vi "获取图像.vi"(1 "确定按钮":bool, 2 "File Path":path=path "C:/labview/labview_小米伺服_CAN总线/种子图片/2.jpeg", 3 "Session In":T1="cam6") -> (0 "Image":T2(plugin-control))   [LabVIEW 2023]
uses:
  <vilib>/userDefined/High Color/IMAQdx.ctl
  <vilib>/vision/driver/NI_Vision_Acquisition_Software.lvlib
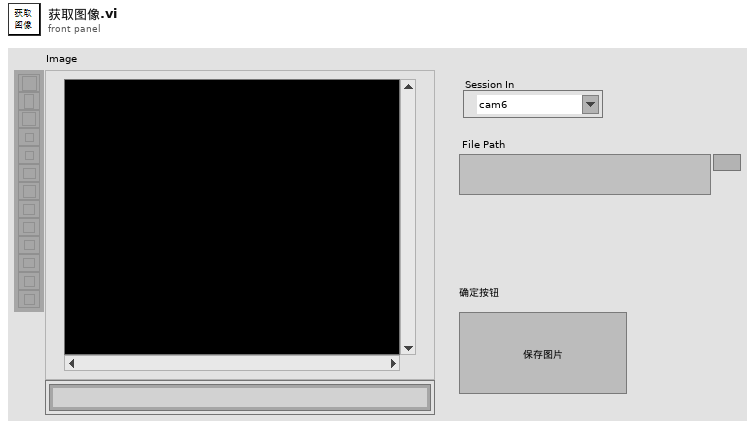
[diagram p1: front panel]
types:
  T1 = typedef "IMAQdx.ctl" = refnum<k21>
  T2 = typedef "IMAQ Image.ctl" = refnum<image>
  T3 = typedef "Image Type" = u32
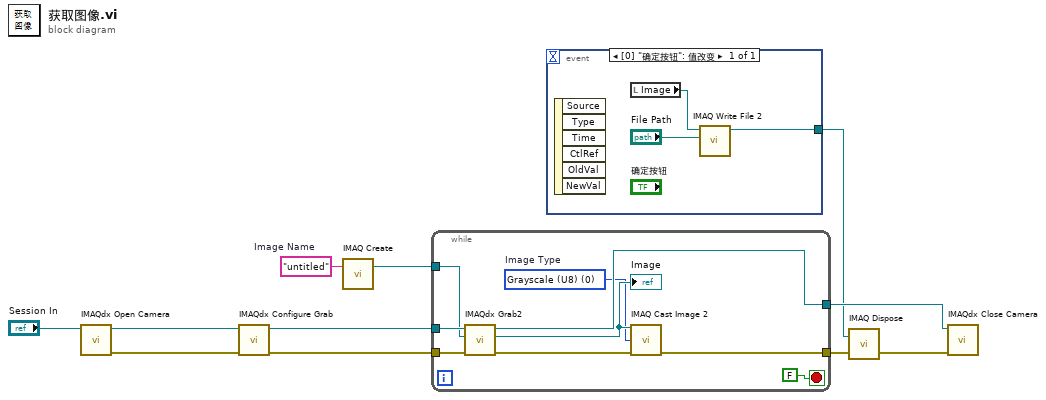
[diagram p0: block diagram]
diagram:
  w11 = "untitled"  # Image Name
  n1 = call <vilib>:"IMAQdx Open Camera.vi"("Session In"="Session In") -> ("error out"=w5:errorcluster, "Session Out"=w6:T1)  [unwired: 9 in]
  n2 = call <vilib>:"IMAQdx Configure Grab.vi"("error in"=w5, "Session In"=w6) -> ("error out"=w8:errorcluster, "Session Out"=w7:T1)  [unwired: 8 in]
  n3 = call "IMAQ Create"("Image Name"=w11) -> ("New Image"=w4:T2)  [unwired: 4 in, 1 out]
  n4 = while {
    tunnel: w8 -> [w19]
    tunnel: w7 -> [w18]
    tunnel: w4 -> [w17]
    tunnel: [w14] -> w3
    tunnel: [w13] -> w2
    stop <- FALSE stop-if-true
    w12 = T3 0 items=["Grayscale (U8)", "Grayscale (I16)", "Grayscale (SGL)", "Complex (CSG)", "RGB (U32)", "HSL (U32)", "RGB (U64)", "Grayscale (U16)"]  # Image Type
    n5 = call <vilib>:"IMAQdx Grab2.vi"("error in"=w19, "Image In"=w17, "Session In"=w18) -> ("error out"=w15:errorcluster, "Image Out"=w16:T2, "Session Out"=w13:T1)  [unwired: 5 in, 1 out]
    "Image" <- w16
    n6 = call "IMAQ Cast Image 2"("Image Src"=w16, "Image Type"=w12, "error in (no error)"=w15) -> ("error out"=w14:errorcluster)  [unwired: 11 in, 1 out]
  }
  n7 = event shown="[0] \"确定按钮\": 值改变" {
    selector: _ -> [_]
    dyn-events: _ -> [_]
    timeout: _ -> [_]
    tunnel: [w21] -> w1
    event "确定按钮": Value Change {
      n8 = event-data() -> ()  [unwired: 1 in, 6 out]
      n9 = local read "Image"() -> (w22:T2)
      n10 = call-poly "IMAQ Write File 2"("File Path"="File Path", "Image"=w22) -> ("Image Out (duplicate)"=w21:T2)  [unwired: 8 in, 1 out]
    }
  }
  n11 = call "IMAQ Dispose"("Image"=w1, "error in (no error)"=w3) -> ("error out"=w10:errorcluster)  [unwired: 4 in]
  n12 = call <vilib>:"IMAQdx Close Camera.vi"("error in"=w10, "Session In"=w2) -> ()  [unwired: 9 in, 1 out]
